vi "Prepare Diagram GObject for Move.vi"(6 "Reference Text to Append (\" Ref\")":string=" Ref", 8 "error in (no error)":errorcluster, 9 "Add as Reference?":bool, 10 "Parsed GObject Class Name":string, 11 "GObject in":refnum<vi>) -> (0 "error out":errorcluster, 1 "Updated Add as Reference?":bool, 2 "Label.Text":string, 3 "GObject out":refnum<vi>)   [LabVIEW 2020, in "Add to Private Data.lvlib"]
uses:
  Add to Private Data.lvlib
  <vilib>/ErrorRing/Error Ring.xnode
  <vilib>/Utility/Data Type/NI_Data Type.lvlib
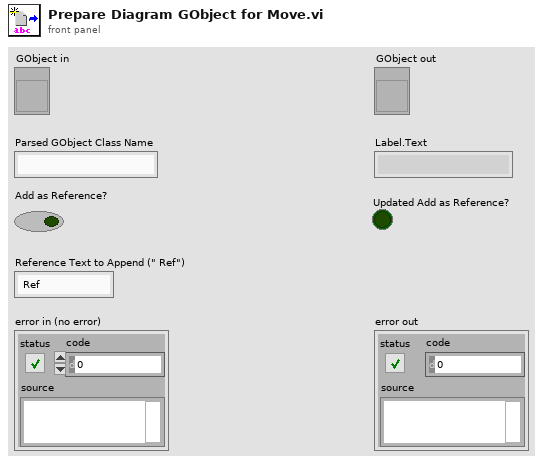
[diagram p1: front panel]
types:
  T1 = typedef "NI_Data Type.lvlib/Data Type.ctl" = enum8{"Invalid Type", "Void", "I8", "I16", "I32", "I64", "U8", "U16", "U32", "U64", "Single Float", "Double Float", "Extended Float", "Single Complex", "Double Complex", "Extended Complex", "Enum U8", "Enum U16", "Enum U32", "Enum U64", "Single Float With Unit", "Double Float With Unit", "Extended Float With Unit", "Single Complex with Unit", "Double Complex with Unit", "Extended Complex with Unit", "Boolean", "String", "Path", "Picture", "Tag", "Array", "Cluster", "Variant", "LV Variant", "Waveform", "Timestamp", "Digital Waveform", "Digital Data", "ExpressData", "Refnum", "External Data", "VI", "Poly VI", "LabVIEW Class Instance", "Fixed Point", "Set Collection", "Map Collection"}
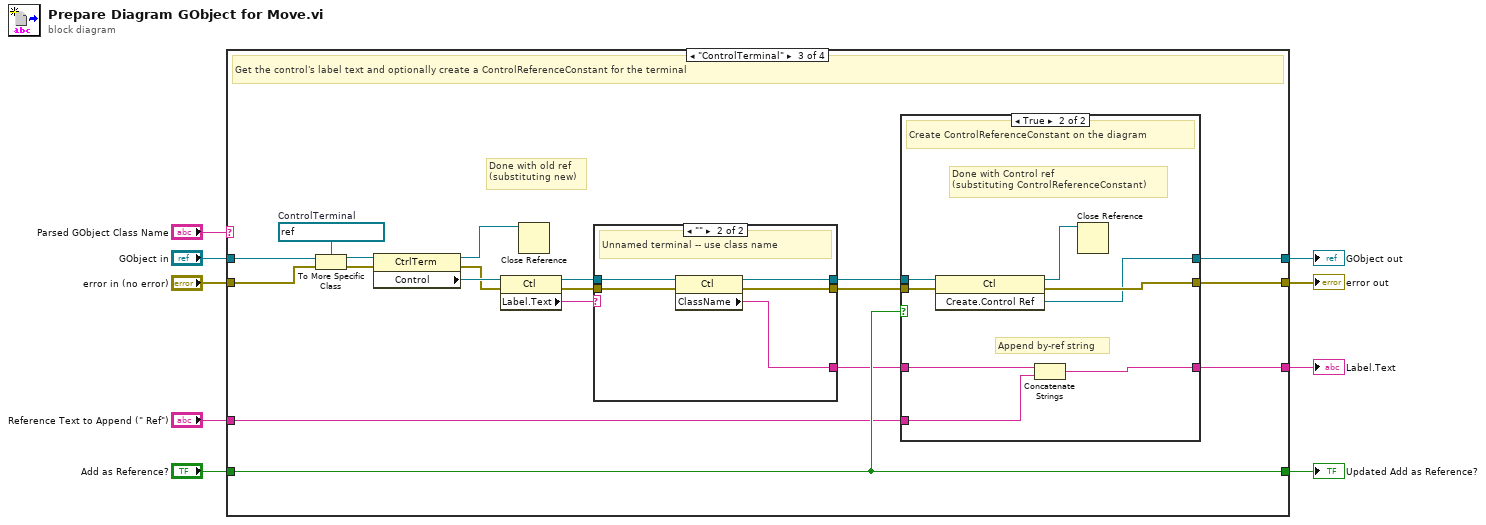
[diagram p0: block diagram]
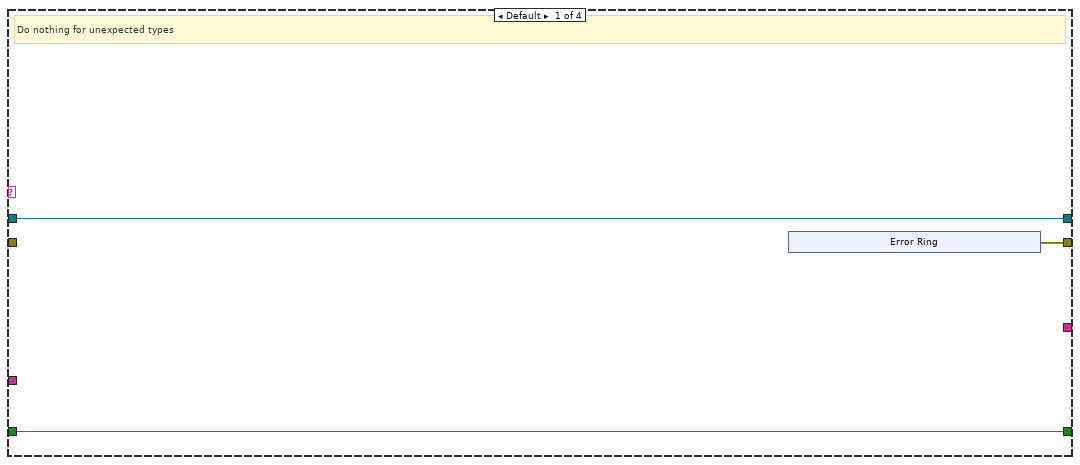
[diagram p2: hidden frame]
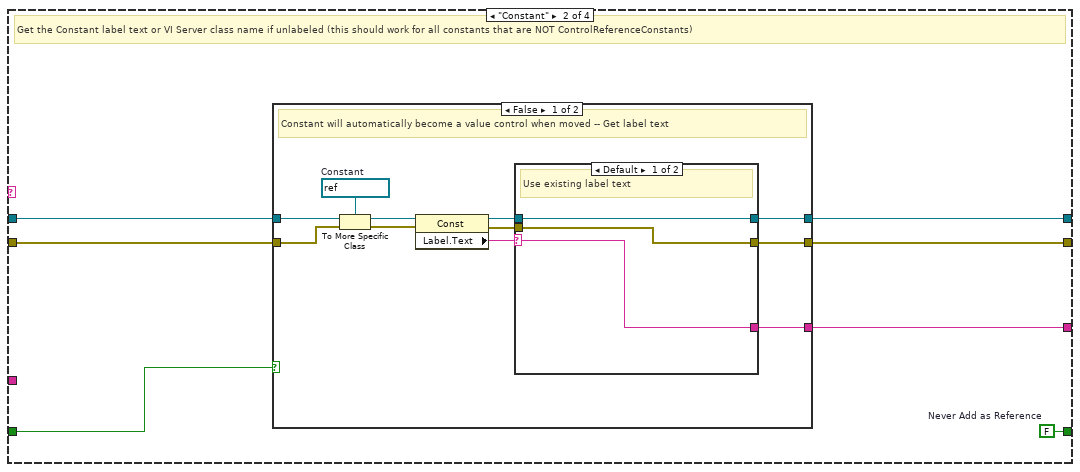
[diagram p3: hidden frame]
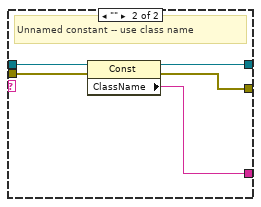
[diagram p4: hidden frame]
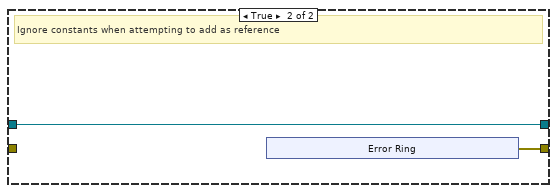
[diagram p5: hidden frame]
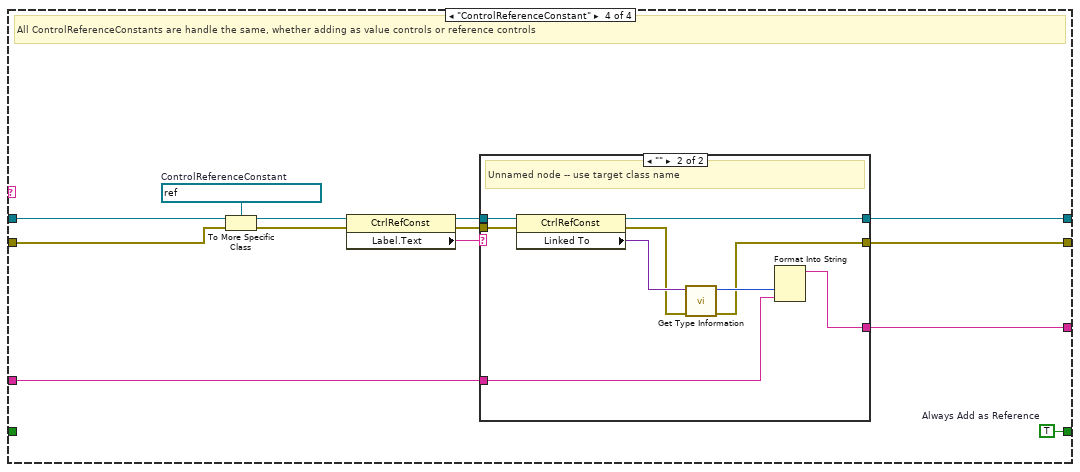
[diagram p8: hidden frame]
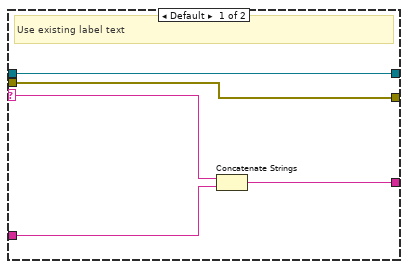
[diagram p9: hidden frame]
diagram:
  n1 = case shown="\"ControlTerminal\"" "Parsed GObject Class Name" {
    tunnel: "GObject in" -> [w12 w20 w57 w91]
    tunnel: "error in (no error)" -> [_ w19 w56 w92]
    tunnel: [_ w15 w44 w83] -> w6
    tunnel: [w12 w18 w55 w85] -> w7
    tunnel: [w11 w17 w61 w84] -> w8
    tunnel: "Add as Reference?" -> [w10 w16 w47 _]
    tunnel: "Reference Text to Append (\" Ref\")" -> [_ _ w43 w82]
    tunnel: [w10 w14 w47 w81] -> w1
    frame Default {
      # "Do nothing for unexpected types"
      n2 = xnode "Error Ring"() -> ("error out"=w11:errorcluster)
    }
    frame "Constant" {
      w14 = FALSE  # Never Add as Reference
      # "Get the Constant label text or VI Server class name if unlabeled (this should work for all constants that are NOT ControlReferenceConstants)"
      n3 = case shown="False" w16 {
        tunnel: w20 -> [w28 w40]
        tunnel: w19 -> [w24 _]
        tunnel: [w22 w40] -> w18
        tunnel: [w21 w41] -> w17
        tunnel: [w25 _] -> w15
        frame False {
          w26 = refnum<vi> refnum  # Constant
          # "Constant will automatically become a value control when moved -- Get label text"
          n4 = To More Specific Class(target class=w26, reference=w28, error in=w24) -> (specific class reference=w27:refnum<vi>, error out=w23:errorcluster)
          n5 = property class="Const"(reference=w27, error in=w23) -> (reference out=w31:refnum<vi>, error out=w30:errorcluster, "Label.Text"=w29:string)
          n6 = case shown="Default" w29 {
            selector: w29 -> [w33 _]
            tunnel: w31 -> [w32 w39]
            tunnel: [w32 w38] -> w22
            tunnel: w30 -> [w34 w37]
            tunnel: [w34 w36] -> w21
            tunnel: [w33 w35] -> w25
            frame Default {
              # "Use existing label text"
            }
            frame "" {
              # "Unnamed constant -- use class name"
              n7 = property class="Const"(reference=w39, error in=w37) -> (reference out=w38:refnum<vi>, error out=w36:errorcluster, "ClassName"=w35:string)
            }
          }
        }
        frame True {
          # "Ignore constants when attempting to add as reference"
          n8 = xnode "Error Ring"() -> ("error out"=w41:errorcluster)
        }
      }
    }
    frame "ControlTerminal" {
      w58 = refnum<vi> refnum  # ControlTerminal
      # "Done with old ref\n(substituting new)"
      # "Get the control's label text and optionally create a ControlReferenceConstant for the terminal"
      n9 = To More Specific Class(target class=w58, reference=w57, error in=w56) -> (specific class reference=w59:refnum<vi>, error out=w60:errorcluster)
      n10 = property class="CtrlTerm"(reference=w59, error in=w60) -> (reference out=w46:refnum<vi>, error out=w50:errorcluster, "Control"=w51:refnum<vi>)
      n11 = property class="Ctl"(reference=w51, error in=w50) -> (reference out=w52:refnum<vi>, error out=w53:errorcluster, "Label.Text"=w54:string)
      n12 = Close Reference(reference=w46) -> ()  [unwired: 1 in, 1 out]
      n13 = case shown="\"\"" w54 {
        selector: w54 -> [w63 _]
        tunnel: w52 -> [w62 w69]
        tunnel: [w62 w68] -> w49
        tunnel: w53 -> [w64 w67]
        tunnel: [w64 w66] -> w48
        tunnel: [w63 w65] -> w45
        frame Default {
          # "Use existing label text"
        }
        frame "" {
          # "Unnamed terminal -- use class name"
          n14 = property class="Ctl"(reference=w69, error in=w67) -> (reference out=w68:refnum<vi>, error out=w66:errorcluster, "ClassName"=w65:string)
        }
      }
      n15 = case shown="True" w47 {
        tunnel: [w72 w80] -> w61
        tunnel: [w71 w79] -> w55
        tunnel: w49 -> [w71 w78]
        tunnel: w48 -> [w72 w77]
        tunnel: w45 -> [w70 w75]
        tunnel: [w70 w74] -> w44
        tunnel: w43 -> [_ w73]
        frame False {
          # "Adding as value control -- do nothing"
        }
        frame True {
          # "Append by-ref string"
          # "Done with Control ref\n(substituting ControlReferenceConstant)"
          # "Create ControlReferenceConstant on the diagram"
          n16 = invoke class="Ctl" method="Create.Control Ref"(reference=w78, error in=w77) -> (reference out=w76:refnum<vi>, error out=w80:errorcluster, "Create Control Ref"=w79:refnum<vi>)  [unwired: 1 in]
          n17 = Concatenate Strings(w75, w73) -> (w74:string)
          n18 = Close Reference(reference=w76) -> ()  [unwired: 1 in, 1 out]
        }
      }
    }
    frame "ControlReferenceConstant" {
      w81 = TRUE  # Always Add as Reference
      w93 = refnum<vi> refnum  # ControlReferenceConstant
      # "All ControlReferenceConstants are handle the same, whether adding as value controls or reference controls"
      n19 = To More Specific Class(target class=w93, reference=w91, error in=w92) -> (specific class reference=w86:refnum<vi>, error out=w87:errorcluster)
      n20 = property class="CtrlRefConst"(reference=w86, error in=w87) -> (reference out=w88:refnum<vi>, error out=w89:errorcluster, "Label.Text"=w90:string)
      n21 = case shown="\"\"" w90 {
        selector: w90 -> [w97 _]
        tunnel: w88 -> [w96 w107]
        tunnel: [w96 w106] -> w85
        tunnel: w89 -> [w98 w105]
        tunnel: [w98 w100] -> w84
        tunnel: [w95 w102] -> w83
        tunnel: w82 -> [w94 w99]
        frame Default {
          # "Use existing label text"
          n22 = Concatenate Strings(w97, w94) -> (w95:string)
        }
        frame "" {
          # "Unnamed node -- use target class name"
          n23 = property class="CtrlRefConst"(reference=w107, error in=w105) -> (reference out=w106:refnum<vi>, error out=w101:errorcluster, "Linked To"=w104:variant)
          n24 = call <vilib>:"Get Type Information.vi"("error in (no error)"=w101, "variant"=w104) -> ("error out"=w100:errorcluster, "type"=w103:T1)  [unwired: 5 in, 3 out]
          n25 = Format Into String(w103, w99) -> (resulting string=w102:string)  [unwired: 3 in, 1 out]
        }
      }
    }
  }
  "error out" <- w8
  "GObject out" <- w7
  "Label.Text" <- w6
  "Updated Add as Reference?" <- w1
